vi "Close Fault Logs.vi"(8 "error in (no error)":errorcluster, 11 "Fault Monitor in":refnum<class "Fault Monitor.lvclass">) -> (0 "error out":errorcluster, 3 "Fault Monitor out":refnum<class "Fault Monitor.lvclass">)   [LabVIEW 2023, in "Fault Monitor.lvlib" / "Fault Monitor.lvclass"]
uses:
  Library/Fault Monitor.lvclass
  Library/Fault Monitor.lvclass/Fault Monitor.ctl
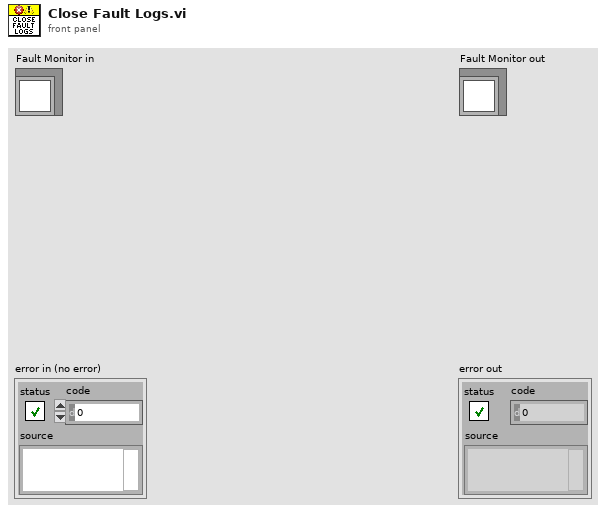
[diagram p1: front panel]
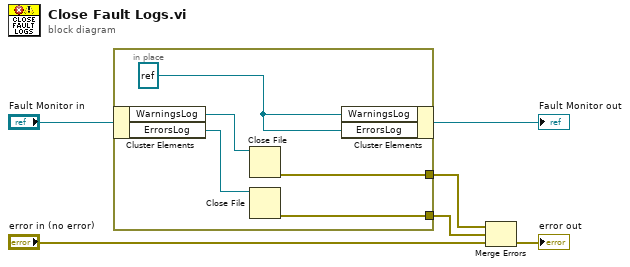
[diagram p0: block diagram]
diagram:
  n1 = in-place {
    in-place-border: [w8] -> w4
    in-place-border: [w7] -> w3
    w11 = refnum<file> refnum ("WarningsLog")
    n2 = in-place-cluster #1("Fault Monitor in") -> ("WarningsLog"=w10:refnum<file>, "ErrorsLog"=w9:refnum<file>)
    n3 = Close File(refnum=w10) -> (error out=w7:errorcluster)  [unwired: 1 in, 1 out]
    n4 = Close File(refnum=w9) -> (error out=w8:errorcluster)  [unwired: 1 in, 1 out]
    n5 = in-place-cluster #1("WarningsLog"=w11, "ErrorsLog"=w11) -> (→"Fault Monitor out":refnum<class "Fault Monitor.lvclass">)
  }
  n6 = Merge Errors(w3, w4, "error in (no error)") -> (→"error out":errorcluster)
